vi "Add Fire Source.vi"(10 "Width":i32, 11 "Pixel Array In":i32[](array[numeric])) -> (3 "Pixel Array Out":i32[](array[numeric]))   [LabVIEW 2019]
doc: "Sets the bottom row of pixels in the buffer to the fire source (element 36 of the palette)."
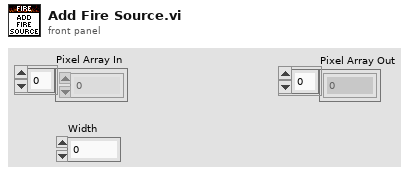
[diagram p1: front panel]
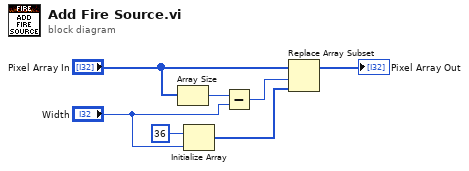
[diagram p0: block diagram]
diagram:
  n1 = Array Size(array="Pixel Array In") -> (size(s)=w5:i32)
  n2 = Initialize Array(36 ("f"), "Width") -> (w6:i32[])
  n3 = Subtract(x=w5, y="Width") -> (x-y=w4:i32)
  n4 = Replace Array Subset(array="Pixel Array In", new element=w6, index=w4) -> (→"Pixel Array Out":i32[])
